vi "MovePos1.vi"(7 "In Contact in":bool, 9 "Move Position 1":bool, 11 "UiDefinition 2":T1) -> (3 "In Contact out":bool)   [LabVIEW 2020]
uses:
  UIReferences.ctl
  C:/Users/User/Desktop/Automation/CurrentVersion/LabviewDXFViewer/bin/Release/LabviewDXFViewer.exe
  LabviewDXFViewer/bin/Release/LabviewDXFViewer.exe
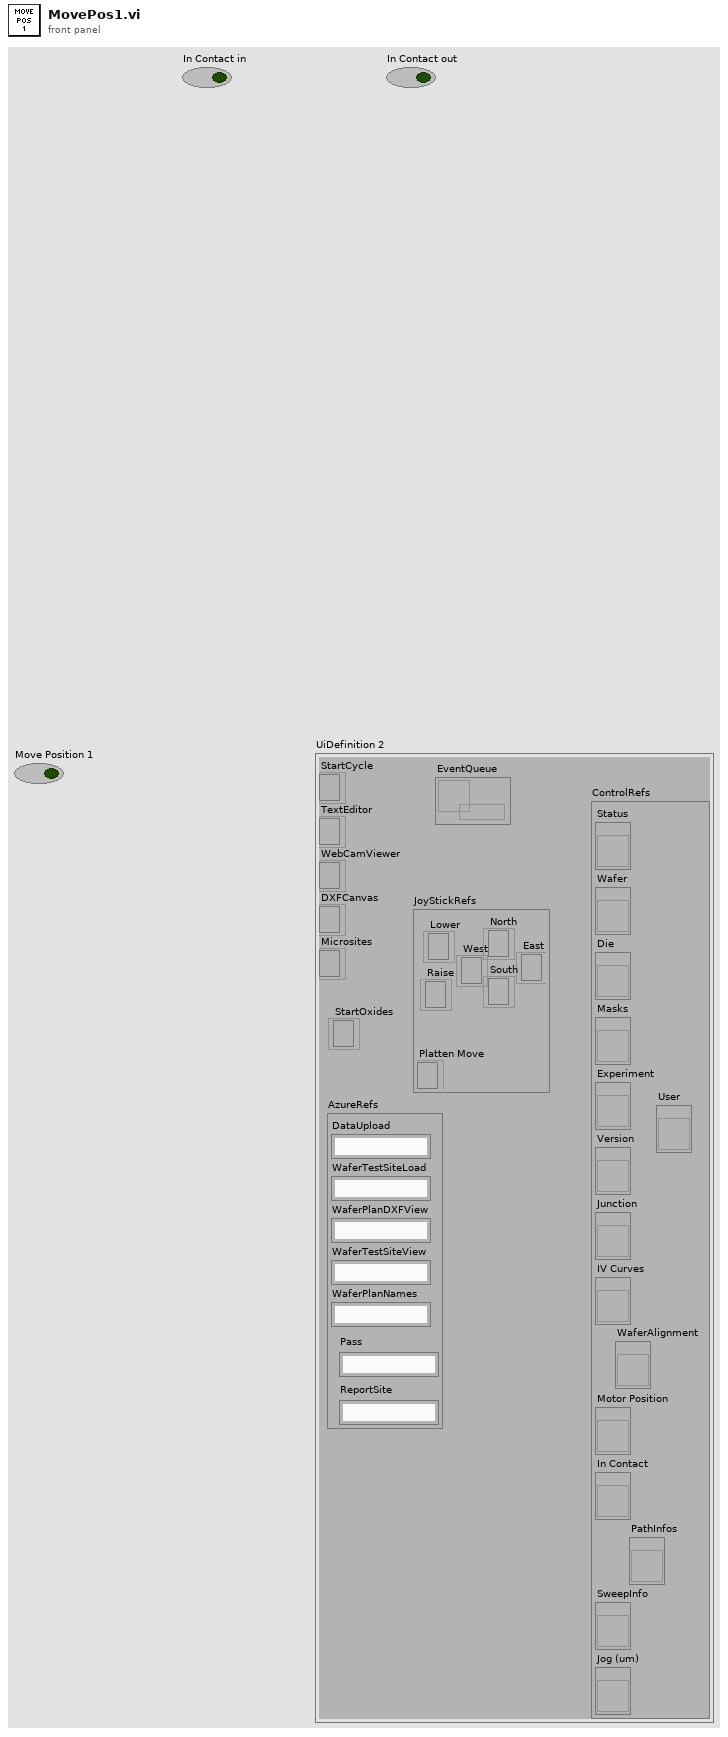
[diagram p1: front panel]
types:
  T1 = typedef "UIReferences.ctl" = cluster{"StartCycle":refnum<k24>, "TextEditor":refnum<k24>, "WebCamViewer":refnum<k24>, "DXFCanvas":refnum<k24>, "Microsites":refnum<k24>, "JoyStickRefs":cluster{"North":refnum<k24>, "Lower":refnum<k24>, "Raise":refnum<k24>, "Platten Move":refnum<k24>, "West":refnum<k24>, "East":refnum<k24>, "South":refnum<k24>}, "AzureRefs":cluster{"DataUpload":string, "WaferTestSiteLoad":string, "WaferPlanDXFView":string, "WaferTestSiteView":string, "WaferPlanNames":string, "Pass":string, "ReportSite":string}, "ControlRefs":cluster{"Status":refnum<vi>, "Wafer":refnum<vi>, "Die":refnum<vi>, "Masks":refnum<vi>, "Experiment":refnum<vi>, "Version":refnum<vi>, "Junction":refnum<vi>, "IV Curves":refnum<vi>, "Motor Position":refnum<vi>, "In Contact":refnum<vi>, "SweepInfo":refnum<vi>, "Jog (um)":refnum<vi>, "PathInfos":refnum<vi>, "User":refnum<vi>, "WaferAlignment":refnum<vi>}, "EventQueue":refnum<queue>, "StartOxides":refnum<k24>}
  T2 = typedef "WaferAlignmentType.ctl" = cluster{"Wafer Units to microns":dbl, "Rotation Misalign":dbl[], "Scale Misalign":dbl, "Steps Per micron":dbl, "Position 1":i32[], "Position 2":i32[], "Lift Distance":i32, "Position 3":i32[], "Jog Height":i32}
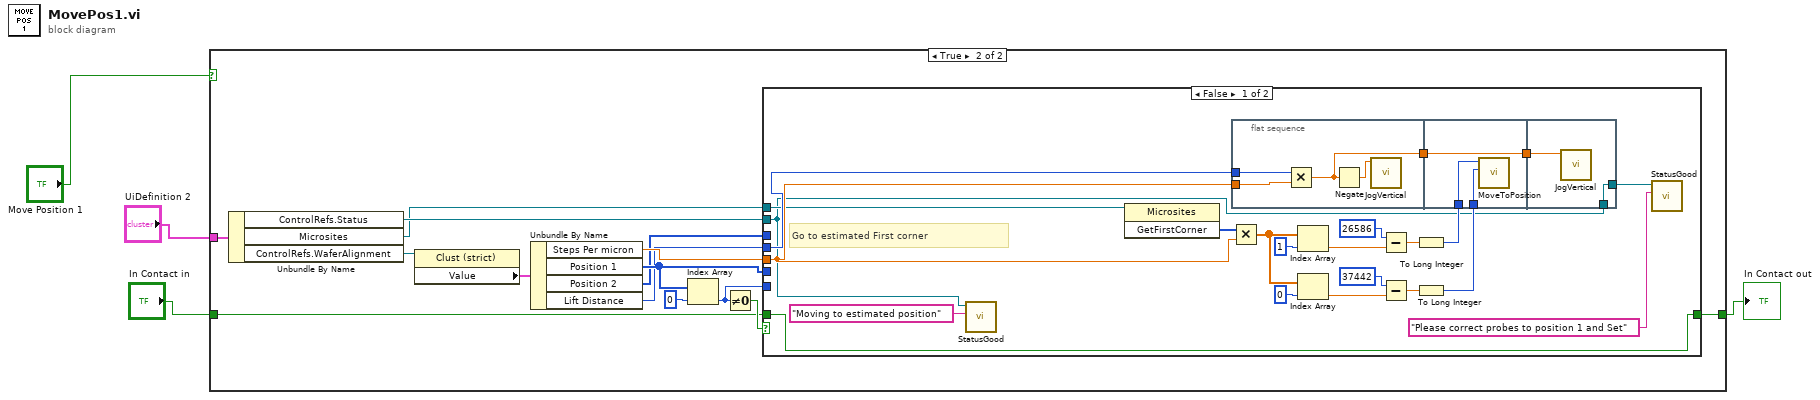
[diagram p0: block diagram]
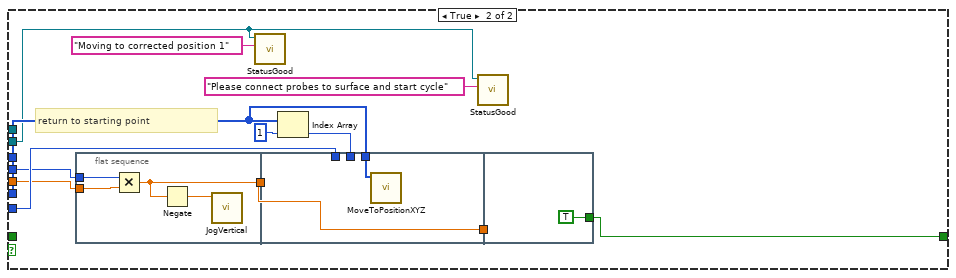
[diagram p3: hidden frame]
diagram:
  n1 = case shown="True" "Move Position 1" {
    tunnel: [w5 w13] -> w3
    tunnel: "In Contact in" -> [w5 w11]
    tunnel: "UiDefinition 2" -> [_ w10]
    frame False {
    }
    frame True {
      n2 = Unbundle By Name(w10) -> ("ControlRefs.Status"=w9:refnum<vi>, "Microsites"=w8:refnum<k24>, "ControlRefs.WaferAlignment"=w7:refnum<vi>)
      n3 = property class="Clust (strict)"(reference=w7) -> ("Value"=w6:T2)  [unwired: 1 in, 2 out]
      n4 = Unbundle By Name(w6) -> ("Steps Per micron"=w16:dbl, "Position 1"=w15:i32[], "Position 2"=w14:i32[], "Lift Distance"=w12:i32)
      n5 = Index Array(array=w15, index=0) -> (element=w17:i32)
      n6 = Not Equal To 0?(x=w17) -> (x != 0?=w18:bool)
      n7 = case shown="False" w18 {
        tunnel: w17 -> [_ w61]
        tunnel: w14 -> [_ _]
        tunnel: w15 -> [_ w55]
        tunnel: w16 -> [w23 w54]
        tunnel: [w22 w53] -> w13
        tunnel: w12 -> [w24 w52]
        tunnel: w11 -> [w22 _]
        tunnel: w8 -> [w21 _]
        tunnel: w9 -> [w20 w51]
        frame False {
          # "Go to estimated First corner"
          n8 = call "StatusGood.vi"("Text.Text"="Moving to estimated position", "String in"=w20) -> ()  [unwired: 10 in]
          n9 = invoke class="Microsites" method="GetFirstCorner"(reference=w21) -> ("GetFirstCorner"=w41:i32[])  [unwired: 2 in, 2 out]
          n10 = Multiply(x=w41, y=w23) -> (x*y=w31:dbl[])
          n11 = flat-sequence {
            tunnel: [w44] -> w33
            tunnel: w23 -> [w43]
            tunnel: w24 -> [w42]
            tunnel: w36 -> [w48]
            tunnel: w35 -> [w47]
            tunnel: [w46] -> w34
            tunnel: w33 -> [w46]
            tunnel: w34 -> [w50]
            tunnel: w20 -> [w49]
            tunnel: [w49] -> w29
            frame #0 {
              n12 = Multiply(x=w42, y=w43) -> (x*y=w44:dbl)
              n13 = Negate(x=w44) -> (-x=w45:dbl)
              n14 = call "JogVertical.vi"("Numeric"=w45) -> ()  [unwired: 11 in]
            }
            frame #1 {
              n15 = call "MoveToPosition.vi"("Y"=w48, "X"=w47) -> ()  [unwired: 10 in]
            }
            frame #2 {
              n16 = call "JogVertical.vi"("Numeric"=w50) -> ()  [unwired: 11 in]
            }
          }
          n17 = Index Array(array=w31, index=1) -> (element=w26:dbl)
          n18 = Index Array(array=w31, index=0) -> (element=w25:dbl)
          n19 = Subtract(x=26586, y=w26) -> (x-y=w38:dbl)
          n20 = Subtract(x=37442, y=w25) -> (x-y=w37:dbl)
          n21 = To Long Integer(number=w38) -> (32bit integer=w35:i32)
          n22 = To Long Integer(number=w37) -> (32bit integer=w36:i32)
          n23 = call "StatusGood.vi"("Text.Text"="Please correct probes to position 1 and Set" ("Status"), "String in"=w29) -> ()  [unwired: 10 in]
        }
        frame True {
          # "return to starting point"
          n24 = flat-sequence {
            tunnel: [w65] -> w58
            tunnel: w54 -> [w64]
            tunnel: w52 -> [w63]
            tunnel: w61 -> [_]
            tunnel: w60 -> [_]
            tunnel: [w68] -> w59
            tunnel: w58 -> [w68]
            tunnel: w55 -> [w67]
            tunnel: w59 -> [_]
            tunnel: [TRUE ("In Contact")] -> w53
            frame #0 {
              n25 = Multiply(x=w63, y=w64) -> (x*y=w65:dbl)
              n26 = Negate(x=w65) -> (-x=w66:dbl)
              n27 = call "JogVertical.vi"("Numeric"=w66) -> ()  [unwired: 11 in]
            }
            frame #1 {
              n28 = call "MoveToPositionXYZ.vi"("Array"=w67) -> ()  [unwired: 11 in]
            }
            frame #2 {
            }
          }
          n29 = call "StatusGood.vi"("Text.Text"="Moving to corrected position 1" ("Status"), "String in"=w51) -> ()  [unwired: 10 in]
          n30 = Index Array(array=w55, index=1) -> (element=w60:i32)
          n31 = call "StatusGood.vi"("Text.Text"="Please connect probes to surface and start cycle" ("Status"), "String in"=w51) -> ()  [unwired: 10 in]
        }
      }
    }
  }
  "In Contact out" <- w3
